vi "Search Optimization.vi"() -> ()   [LabVIEW 2017, in "Tree API.lvlib" / "Tree.lvclass"]
uses:
  Tree.lvclass
panel:
  out "Results Valid":bool=TRUE
  out "Impr. minus Optimization Time":dbl=0.0933169201889541 format="%#.1p"
  out "Speed Improvement":dbl=0.09704901871737093 format="%#.1p"
  out "Creation Time":dbl=0.002733134519075975 format="%#.1p"
  out "UI Drawing Time":dbl=0.034517327236244455 format="%#.1p"
  out "Unoptimized Search":dbl=0.09730149249662645 format="%#.1p"
  out "Optimization Time":dbl=0.0037320985284168273 format="%#.1p"
  out "Optimized Search":dbl=0.0002524737792555243 format="%#.1p"
  out "# Search Paths":i32=125
  in  "Tree":string(tree)="Root"
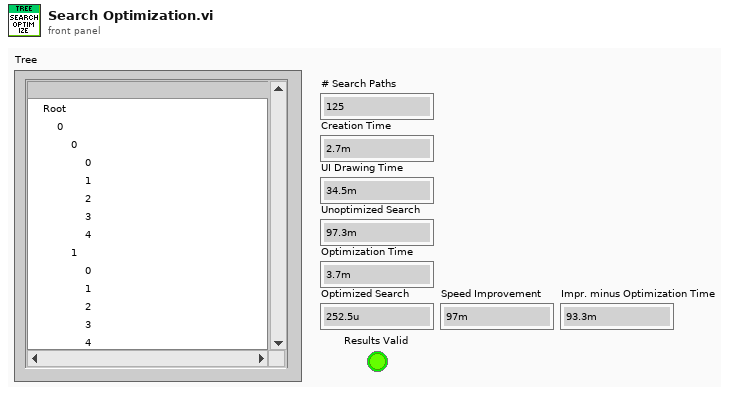
[diagram p1: front panel]
types:
  T1 = cluster{"Left Cell String":string, "Child Text":string[], "Child Tag":string, "Item Indent":i32, "Child Only?":bool, "Glyph Index":i32}[]
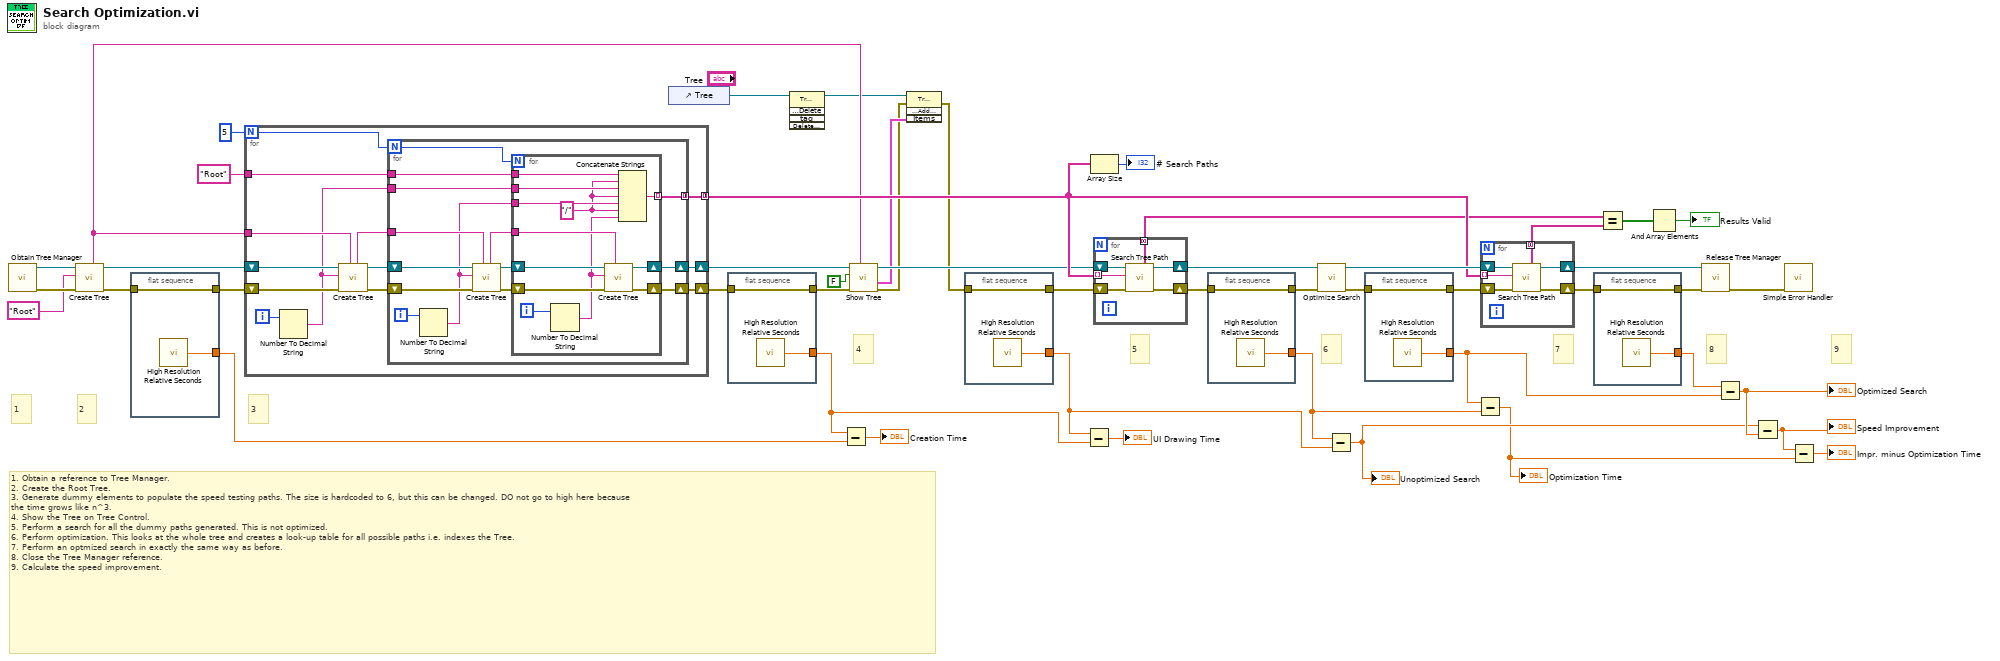
[diagram p0: block diagram]
diagram:
  # "1. Obtain a reference to Tree Manager.\n2. Create the Root Tree.\n3. Generate dummy elements to populate the speed testing paths. The size is hardcoded to 6, but this can be changed. DO not go to high here because\nthe time grows like n^3.\n4. Show the Tree on Tree Control.\n5. Perform a search for all the dummy paths generated. This is not optimized.\n6. Perform optimization. This looks at the whole tree and creates a look-up table for all possible paths i.e. indexes the Tree.\n7. Perform an optmized search in exactly the same way as before.\n8. Close the Tree Manager reference.\n9. Calculate the speed improvement."
  # "9"
  # "8"
  # "7"
  # "6"
  # "5"
  # "4"
  # "3"
  # "2"
  # "1"
  n1 = call "Obtain Tree Manager.vi"() -> ("Error Out"=w48:errorcluster, "Tree"=w49:refnum<data-value>)  [unwired: 10 in]
  n2 = call "Create Tree.vi"("Error In"=w48, "Name"="Root", "Tree Manager"=w49) -> ("Error Out"=w43:errorcluster, "Tree Manager"=w45:refnum<data-value>, "Unique ID"=w12:string)  [unwired: 6 in]
  n3 = flat-sequence {
    tunnel: [w51] -> w44
    tunnel: w43 -> [w51]
    tunnel: [w50] -> w26
    frame #0 {
      n4 = call <vilib>:"High Resolution Relative Seconds.vi"() -> ("relative seconds"=w50:dbl)
    }
  }
  n5 = for {
    N: 5 -> [w55]
    shift-right: [w57] -> w24
    shift-left: w45 -> [w64]
    shift-right: [w56] -> w22
    shift-left: w44 -> [w63]
    tunnel: w12 -> [w62]
    tunnel: "Root" ("Name") -> [w54]
    tunnel: [w52] -> w20 mode=concatenating
    i -> [w61]
    n6 = Number To Decimal String(number=w61) -> (decimal integer string=w53:string)  [unwired: 1 in]
    n7 = call "Create Tree.vi"("Parent ID (empty)"=w62, "Error In"=w63, "Name"=w53, "Tree Manager"=w64) -> ("Error Out"=w58:errorcluster, "Tree Manager"=w60:refnum<data-value>, "Unique ID"=w59:string)  [unwired: 5 in]
    n8 = for {
      N: w55 -> [w71]
      shift-right: [w70] -> w57
      shift-left: w60 -> [w78]
      tunnel: w59 -> [w77]
      shift-right: [w69] -> w56
      shift-left: w58 -> [w75]
      tunnel: w54 -> [w68]
      tunnel: w53 -> [w67]
      tunnel: [w65] -> w52 mode=concatenating
      i -> [w76]
      n9 = Number To Decimal String(number=w76) -> (decimal integer string=w66:string)  [unwired: 1 in]
      n10 = call "Create Tree.vi"("Parent ID (empty)"=w77, "Error In"=w75, "Name"=w66, "Tree Manager"=w78) -> ("Error Out"=w72:errorcluster, "Tree Manager"=w74:refnum<data-value>, "Unique ID"=w73:string)  [unwired: 5 in]
      n11 = for {
        N: w71 -> [_]
        tunnel: w73 -> [w88]
        shift-right: [w85] -> w69
        shift-left: w72 -> [w87]
        shift-right: [w86] -> w70
        shift-left: w74 -> [w89]
        tunnel: w68 -> [w84]
        tunnel: w67 -> [w83]
        tunnel: w66 -> [w82]
        tunnel: [w79] -> w65 mode=indexing
        i -> [w90]
        w81 = "/" ("string")
        n12 = Number To Decimal String(number=w90) -> (decimal integer string=w80:string)  [unwired: 1 in]
        n13 = call "Create Tree.vi"("Parent ID (empty)"=w88, "Error In"=w87, "Name"=w80, "Tree Manager"=w89) -> ("Error Out"=w85:errorcluster, "Tree Manager"=w86:refnum<data-value>)  [unwired: 5 in, 1 out]
        n14 = Concatenate Strings(w84, w81, w83, w81, w82, w81, w80) -> (w79:string)
      }
    }
  }
  n15 = control-ref of="Tree"() -> (w4:refnum<vi>)
  n16 = flat-sequence {
    tunnel: [w92] -> w42
    tunnel: w22 -> [w92]
    tunnel: [w91] -> w14
    frame #0 {
      n17 = call <vilib>:"High Resolution Relative Seconds.vi"() -> ("relative seconds"=w91:dbl)
    }
  }
  n18 = invoke class="Tree (strict)" method="Edit Tree Items.Delete"(reference=w4) -> (reference out=w5:refnum<vi>)  [unwired: 4 in, 4 out]
  n19 = Subtract(x=w14, y=w26) -> (x-y=→"Creation Time":dbl)
  n20 = call "Show Tree.vi"("Root ID"=w12, "Error In"=w42, "Show IDs (False)"=FALSE ("Show IDs (True)"), "Tree"=w24) -> ("Error Out"=w2:errorcluster, "Items Out"=w3:T1, "Tree"=w13:refnum<data-value>)  [unwired: 5 in]
  n21 = invoke class="Tree (strict)" method="Edit Tree Items.Add Multiple Items to End"(reference=w5, error in=w2, "Items"=w3) -> (error out=w1:errorcluster)  [unwired: 1 in, 3 out]
  n22 = flat-sequence {
    tunnel: [w94] -> w41
    tunnel: w1 -> [w94]
    tunnel: [w93] -> w23
    frame #0 {
      n23 = call <vilib>:"High Resolution Relative Seconds.vi"() -> ("relative seconds"=w93:dbl)
    }
  }
  n24 = Subtract(x=w23, y=w14) -> (x-y=→"UI Drawing Time":dbl)
  n25 = Array Size(array=w20) -> (size(s)=→"# Search Paths":i32)
  n26 = for {
    shift-right: [w97] -> w37
    shift-left: w13 -> [w100]
    shift-right: [w98] -> w40
    shift-left: w41 -> [w99]
    tunnel: w20 -> [w96] mode=indexing
    tunnel: [w95] -> w9 mode=concatenating
    n27 = call "Search Tree Path.vi"("Error In"=w99, "Tree Path"=w96, "Tree Manager"=w100) -> ("Error Out"=w98:errorcluster, "Tree Manager"=w97:refnum<data-value>, "Tree IDs"=w95:string[])  [unwired: 6 in]
  }
  n28 = flat-sequence {
    tunnel: [w102] -> w38
    tunnel: w40 -> [w102]
    tunnel: [w101] -> w28
    frame #0 {
      n29 = call <vilib>:"High Resolution Relative Seconds.vi"() -> ("relative seconds"=w101:dbl)
    }
  }
  n30 = call "Optimize Search.vi"("Error In"=w38, "Tree Manager"=w37) -> ("Error Out"=w36:errorcluster, "Tree Manager"=w34:refnum<data-value>)  [unwired: 8 in]
  n31 = Subtract(x=w28, y=w23) -> (x-y=w18:dbl)
  "Unoptimized Search" <- w18
  n32 = flat-sequence {
    tunnel: [w104] -> w35
    tunnel: w36 -> [w104]
    tunnel: [w103] -> w29
    frame #0 {
      n33 = call <vilib>:"High Resolution Relative Seconds.vi"() -> ("relative seconds"=w103:dbl)
    }
  }
  n34 = Subtract(x=w29, y=w28) -> (x-y=w15:dbl)
  "Optimization Time" <- w15
  n35 = for {
    shift-right: [w107] -> w32
    shift-left: w34 -> [w110]
    shift-right: [w108] -> w33
    shift-left: w35 -> [w109]
    tunnel: w20 -> [w106] mode=indexing
    tunnel: [w105] -> w8 mode=concatenating
    n36 = call "Search Tree Path.vi"("Error In"=w109, "Tree Path"=w106, "Tree Manager"=w110) -> ("Error Out"=w108:errorcluster, "Tree Manager"=w107:refnum<data-value>, "Tree IDs"=w105:string[])  [unwired: 6 in]
  }
  n37 = flat-sequence {
    tunnel: [w112] -> w31
    tunnel: w33 -> [w112]
    tunnel: [w111] -> w30
    frame #0 {
      n38 = call <vilib>:"High Resolution Relative Seconds.vi"() -> ("relative seconds"=w111:dbl)
    }
  }
  n39 = Equal?(x=w9, y=w8) -> (x = y?=w11:bool[])
  n40 = And Array Elements(Boolean array=w11) -> (logical AND=→"Results Valid":bool)
  n41 = call "Release Tree Manager.vi"("Error In"=w31, "Tree"=w32) -> ("Error Out"=w7:errorcluster)  [unwired: 9 in]
  n42 = Subtract(x=w30, y=w29) -> (x-y=w19:dbl)
  "Optimized Search" <- w19
  n43 = Subtract(x=w18, y=w19) -> (x-y=w17:dbl)
  "Speed Improvement" <- w17
  n44 = call <vilib>:"Simple Error Handler.vi"("error in (no error)"=w7) -> ()  [unwired: 4 in, 5 out]
  n45 = Subtract(x=w17, y=w15) -> (x-y=→"Impr. minus Optimization Time":dbl)
